vi "Get ID.vi"(8 "error in (no error)":errorcluster, 11 "Handle in":i32) -> (0 "error out":errorcluster, 2 "ID":string, 3 "Handle out":i32)   [LabVIEW 2013, in "Thorlabs_MC2000B.lvlib"]
uses:
  <instrlib>/Thorlabs_MC2000B/Thorlabs_MC2000B.lvlib
  <instrlib>/Thorlabs_MC2000B/Library/MC2000CommandLibWin32.dll
  Program Files/National Instruments/LabVIEW 2011/instr.lib/Thorlabs_MC2000B/Library/MC2000CommandLibWin64.dll
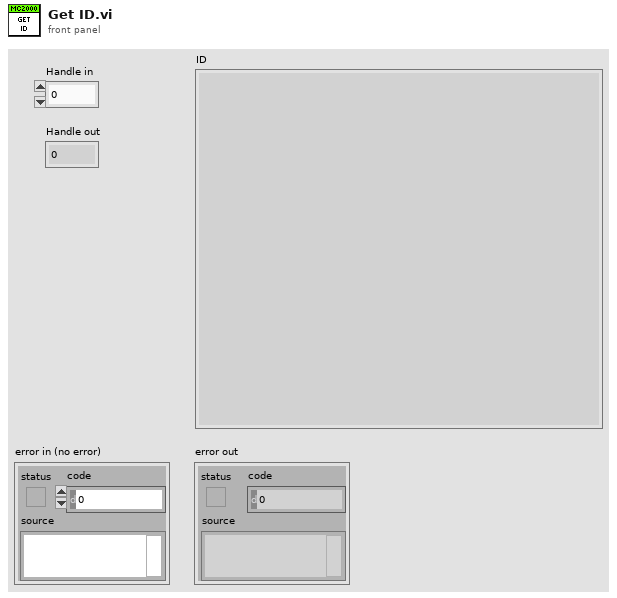
[diagram p1: front panel]
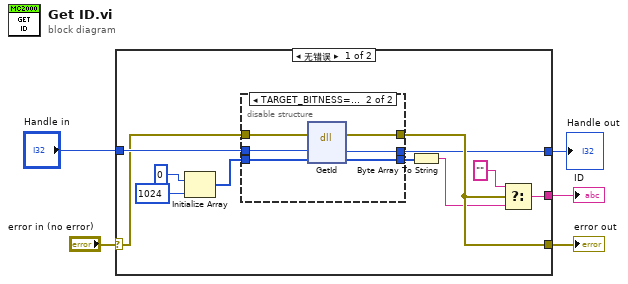
[diagram p0: block diagram]
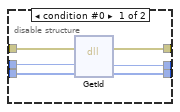
[diagram p2: hidden frame]
diagram:
  n1 = case shown="无错误" "error in (no error)" {
    selector: "error in (no error)" -> [w6 w30]
    tunnel: [w16 w30] -> w5
    tunnel: [w14 _] -> w4
    tunnel: "Handle in" -> [w13 w29]
    tunnel: [w12 w29] -> w1
    frame No Error {
      n2 = Initialize Array(u8 0, 1024 ("dimension size")) -> (w9:u8[])
      n3 = disable-structure shown="TARGET_BITNESS==32" {
        disable-tunnel: [w22 w28] -> w16
        disable-tunnel: w13 -> [w21 w27]
        disable-tunnel: [w20 w26] -> w12
        disable-tunnel: w9 -> [w19 w25]
        disable-tunnel: [w18 w24] -> w8
        disable-tunnel: w6 -> [w17 w23]
        frame condition #0 {
          n4 = dll-call lib="D:/Program Files/National Instruments/LabVIEW 2011/instr.lib/Thorlabs_MC2000B/Library/MC2000CommandLibWin64.dll" fn="GetId"(error in=w17, "handle"=w21, "ID"=w19) -> (error out=w22:errorcluster, "handle"=w20:i32, "ID"=w18:u8[])  [unwired: 3 in, 1 out]
        }
        frame condition #1 (active) {
          n5 = dll-call lib="C:/Program Files (x86)/National Instruments/LabVIEW 2013/instr.lib/Thorlabs_MC2000B/Library/MC2000CommandLibWin32.dll" fn="GetId"(error in=w23, "handle"=w27, "ID"=w25) -> (error out=w28:errorcluster, "handle"=w26:i32, "ID"=w24:u8[])  [unwired: 3 in, 1 out]
        }
      }
      n6 = Byte Array To String(unsigned byte array=w8) -> (string=w7:string)
      n7 = Select(t="", s=w16, f=w7) -> (s? t:f=w14:string)
    }
    frame Error {
    }
  }
  "error out" <- w5
  "ID" <- w4
  "Handle out" <- w1
